vi "Initialize Transfer Groups.vi"(8 "error in (no error)":errorcluster, 10 "Transfer Groups Configurations":T1[](array[typedef]) {"transfers"."channels"."string offset" format="%d bytes"}, 11 "PXImc Transceiver in":refnum<class "PXImc Transceiver.lvclass">) -> (0 "error out":errorcluster, 3 "PXImc Transceiver out":refnum<class "PXImc Transceiver.lvclass">)   [LabVIEW 2017, in "PXImc.lvlib" / "PXImc Transceiver.lvclass"]
uses:
  PXImc Transceiver.lvclass
  Builds/Data Sharing Framework/Current/Core/DSF Core.lvlibp/Typedefs/DSF Engine Transfer Group Configuration.ctl
  Builds/Data Sharing Framework/Current/Core/DSF Core.lvlibp/Typedefs/DSF Direction.ctl
  Builds/Data Sharing Framework/Current/Core/DSF Core.lvlibp/Typedefs/DSF Timing Info.ctl
  Builds/Data Sharing Framework/Current/Core/DSF Core.lvlibp/Typedefs/DSF Settings Info.ctl
  Builds/Data Sharing Framework/Current/Core/DSF Core.lvlibp/Typedefs/DSF Engine Transfer Configuration.ctl
  Builds/Data Sharing Framework/Current/Core/DSF Core.lvlibp/Typedefs/DSF Byte Order.ctl
  Builds/Data Sharing Framework/Current/Core/DSF Core.lvlibp/Typedefs/DSF Engine Channel Configuration.ctl
  Builds/Data Sharing Framework/Current/Core/DSF Core.lvlibp/Typedefs/DSF Data Type.ctl
  Builds/Data Sharing Framework/Current/Core/DSF Core.lvlibp/Typedefs/DSF Timeout Behavior.ctl
  PXImc Group Data.ctl
  PXImc Transfer Data.ctl
  PXImc Transceiver.lvclass/PXImc Transceiver.ctl
  Builds/Data Sharing Framework/Current/Core/DSF Core.lvlibp
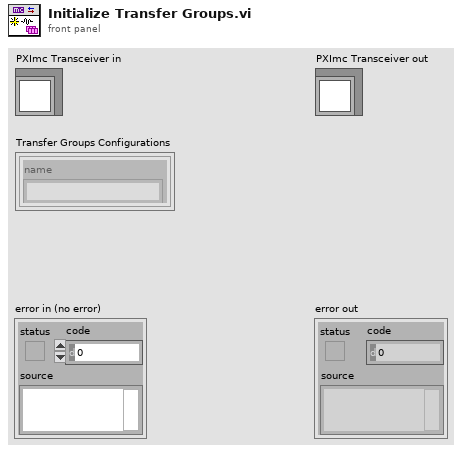
[diagram p1: front panel]
types:
  T1 = typedef "DSF Core.lvlibp/DSF Engine Transfer Group Configuration.ctl" = cluster{"name":string, "direction":T2, "cycle timing":T3, "thread index":i32, "settings":T4, "transfers":T5[], "timeout behavior":T9}
  T2 = typedef "DSF Core.lvlibp/DSF Direction.ctl" = enum8{"Tx", "Rx"}
  T3 = typedef "DSF Core.lvlibp/DSF Timing Info.ctl" = cluster{"priority":u64, "decimation":u64, "offset":u64}
  T4 = typedef "DSF Core.lvlibp/DSF Settings Info.ctl" = cluster{"component":string, "name":string, "values":cluster{"key":string, "value":string}[]}[]
  T5 = typedef "DSF Core.lvlibp/DSF Engine Transfer Configuration.ctl" = cluster{"name":string, "byte order":T6, "settings":T4, "channels":T7[]}
  T6 = typedef "DSF Core.lvlibp/DSF Byte Order.ctl" = enum8{"big-endian", "little-endian"}
  T7 = typedef "DSF Core.lvlibp/DSF Engine Channel Configuration.ctl" = cluster{"string offset":u64, "name":string, "units":string, "engine data type":T8, "string data type":T8, "settings":T4}
  T8 = typedef "DSF Core.lvlibp/DSF Data Type.ctl" = enum8{"Bool", "SGL", "DBL", "I8", "I16", "I32", "I64", "U8", "U16", "U32", "U64"}
  T9 = typedef "DSF Core.lvlibp/DSF Timeout Behavior.ctl" = enum8{"Increment Late Count", "Throw Error"}
  T10 = typedef "PXImc.lvlib/PXImc Transceiver.lvclass/PXImc Group Data.ctl" = cluster{"direction":T2, "transfers":T11[]}
  T11 = typedef "PXImc.lvlib/PXImc Transceiver.lvclass/PXImc Transfer Data.ctl" = cluster{"stream id":u16, "session":refnum<k21>}
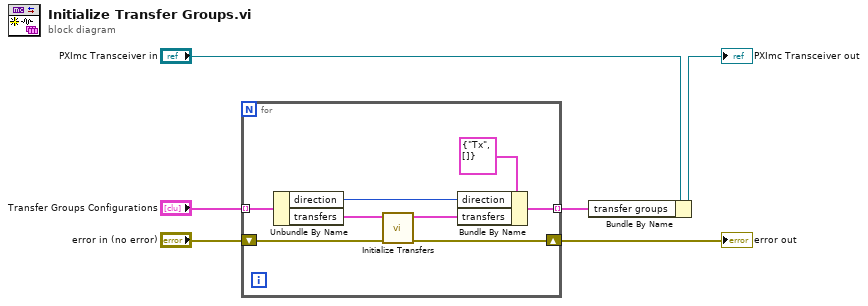
[diagram p0: block diagram]
diagram:
  n1 = for {
    tunnel: "Transfer Groups Configurations" -> [w13] mode=indexing
    tunnel: [w10] -> w3 mode=indexing
    shift-right: [w9] -> w4
    shift-left: "error in (no error)" -> [w8]
    n2 = Unbundle By Name(w13) -> ("direction"=w11:T2, "transfers"=w14:T5[])
    n3 = call "Initialize Transfers.vi"("error in (no error)"=w8, "transfer configurations"=w14) -> ("error out"=w9:errorcluster, "transfers"=w7:T11[])  [unwired: 8 in]
    n4 = Bundle By Name(cluster=T10 {"direction"=enum."Tx", "transfers"=[]} ("PXImc Transfer"), "direction"=w11, "transfers"=w7) -> (w10:T10)
  }
  "error out" <- w4
  n5 = Bundle By Name(cluster="PXImc Transceiver in", "transfer groups"=w3) -> (→"PXImc Transceiver out":refnum<class "PXImc Transceiver.lvclass">)
